vi "Clean Wave.vi"(6 "line clock out":i32, 7 "Galvo signal in":u32, 8 "pixel clock_pulse width in":i32, 9 "Clean wave":bool, 10 "Address counter output":u32, 11 "Galvo signal readed out":u32) -> (0 "Address counter":u32, 1 "Galvo signal readed out":u32, 2 "Galvo signal in":u32, 3 "line clock":i32, 5 "pixel clock_pulse width out":i32)   [LabVIEW 2015]
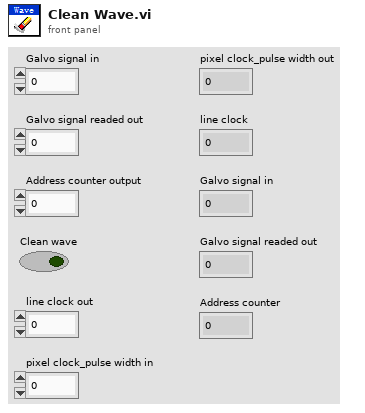
[diagram p1: front panel]
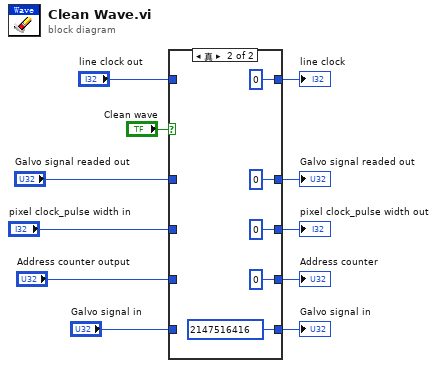
[diagram p0: block diagram]
diagram:
  n1 = case shown="真" "Clean wave" {
    tunnel: "Galvo signal in" -> [w16 _]
    tunnel: [w16 u32 2147516416 ("Galvo signal")] -> w6
    tunnel: [w15 u32 0 ("Galvo signal readed")] -> w7
    tunnel: "Galvo signal readed out" -> [w15 _]
    tunnel: [w14 0] -> w9
    tunnel: "pixel clock_pulse width in" -> [w14 _]
    tunnel: [w13 u32 0 ("Address counter")] -> w10
    tunnel: "Address counter output" -> [w13 _]
    tunnel: [w12 0 ("line clock")] -> w8
    tunnel: "line clock out" -> [w12 _]
    frame False {
    }
    frame True {
    }
  }
  "Address counter" <- w10
  "pixel clock_pulse width out" <- w9
  "line clock" <- w8
  "Galvo signal readed out" <- w7
  "Galvo signal in" <- w6
